vi "Script_DuplicateCDS.vi"() -> ()   [LabVIEW 2024]
panel:
  out "Conditions":string[](array[string])
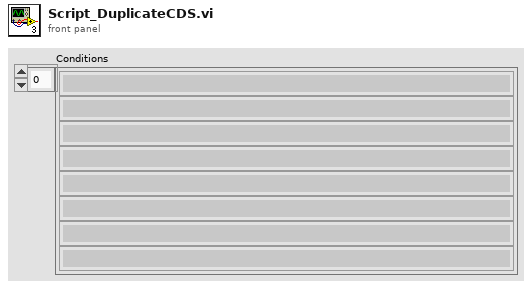
[diagram p1: front panel]
types:
  T1 = enum32{"Conditional Disable Style", "Diagram Disable Style", "Type Specialization Style"}
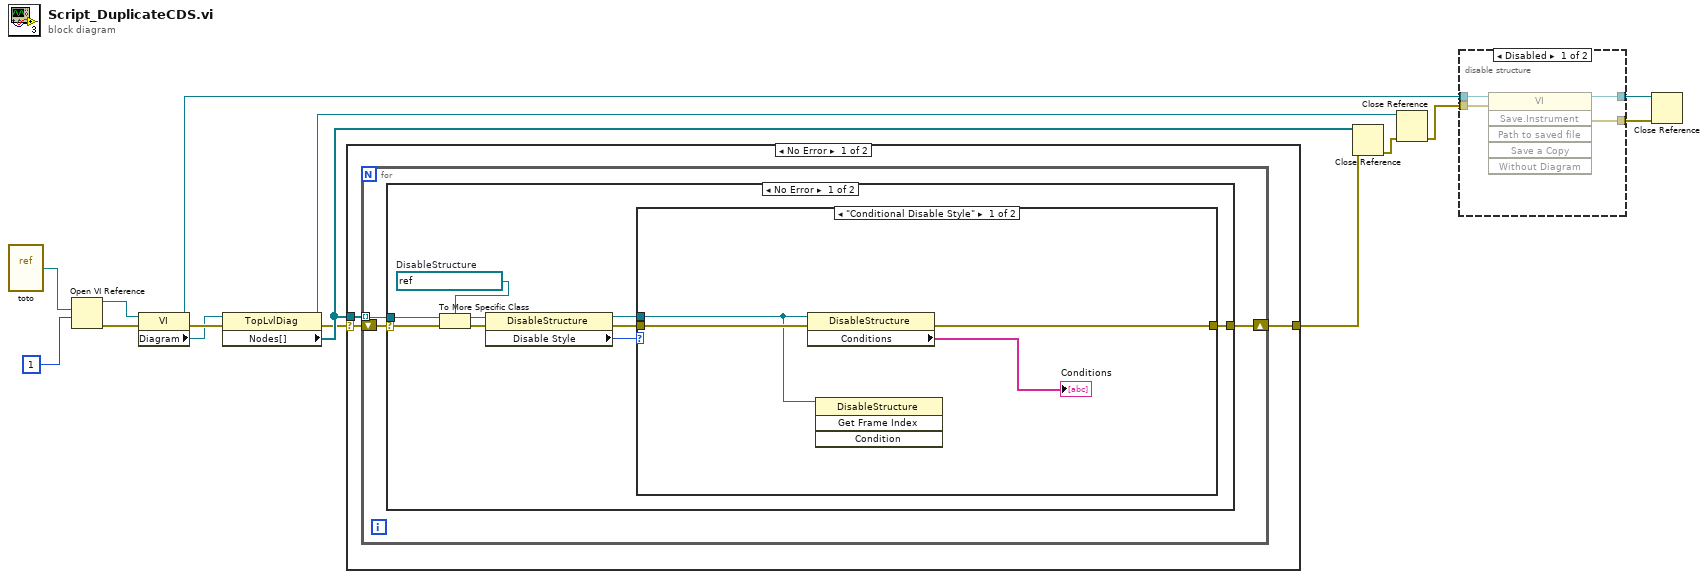
[diagram p0: block diagram]
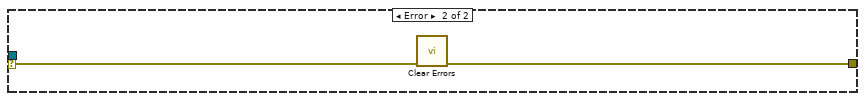
[diagram p4: hidden frame]
diagram:
  n1 = vi-ref "toto.vi"() -> (w15:refnum<vi>)
  n2 = Open VI Reference(vi path=w15, options=1) -> (vi reference=w12:refnum<vi>, error out=w13:errorcluster)  [unwired: 4 in]
  n3 = property class="VI"(reference=w12, error in=w13) -> (reference out=w5:refnum<vi>, error out=w11:errorcluster, "Diagram"=w7:refnum<vi>)
  n4 = property class="TopLvlDiag"(reference=w7, error in=w11) -> (reference out=w10:refnum<vi>, error out=w1:errorcluster, "Nodes[]"=w3:refnum<vi>[])
  n5 = case shown="No Error" w1 {
    selector: w1 -> [w16 w38]
    tunnel: w3 -> [w18 _]
    tunnel: [w17 w38] -> w2
    frame No Error {
      n6 = for {
        tunnel: w18 -> [w20] mode=indexing
        shift-right: [w19] -> w17
        shift-left: w16 -> [w21]
        n7 = case shown="No Error" w21 {
          selector: w21 -> [w30 w37]
          tunnel: w20 -> [w28 _]
          tunnel: [w23 w36] -> w19
          frame No Error {
            w27 = refnum<vi> refnum  # DisableStructure
            n8 = To More Specific Class(target class=w27, reference=w28, error in=w30) -> (specific class reference=w26:refnum<vi>, error out=w29:errorcluster)
            n9 = property class="DisableStructure"(reference=w26, error in=w29) -> (reference out=w22:refnum<vi>, error out=w25:errorcluster, "Disable Style"=w24:T1)
            n10 = case shown="\"Conditional Disable Style\"" w24 {
              tunnel: w25 -> [w34 w35]
              tunnel: [w33 w35] -> w23
              tunnel: w22 -> [w31 _]
              frame "Conditional Disable Style" {
                n11 = property class="DisableStructure"(reference=w31, error in=w34) -> (error out=w33:errorcluster, "Conditions"=→"Conditions":string[])  [unwired: 1 out]
                n12 = invoke class="DisableStructure" method="Get Frame Index"(reference=w31) -> ()  [unwired: 3 in, 4 out]
              }
              frame Default {
              }
            }
          }
          frame Error {
            n13 = call <vilib>:"Clear Errors.vi"("error in (no error)"=w37) -> ("error out"=w36:errorcluster)  [unwired: 5 in, 1 out]
          }
        }
      }
    }
    frame Error {
    }
  }
  n14 = Close Reference(reference=w3, error in (no error)=w2) -> (error out=w9:errorcluster)
  n15 = Close Reference(reference=w10, error in (no error)=w9) -> (error out=w8:errorcluster)
  n16 = disable-structure shown="Disabled" {
    disable-tunnel: w8 -> [w42 w44]
    disable-tunnel: [w41 w44] -> w6
    disable-tunnel: w5 -> [w40 w43]
    disable-tunnel: [w39 w43] -> w4
    frame Disabled {
      n17 = invoke class="VI" method="Save.Instrument"(reference=w40, error in=w42) -> (reference out=w39:refnum<vi>, error out=w41:errorcluster)  [unwired: 4 in, 4 out]
    }
    frame Enabled {
    }
  }
  n18 = Close Reference(reference=w4, error in (no error)=w6) -> ()  [unwired: 1 out]
